vi "Get Semaphore.vi"(4 "error in":errorcluster, 7 "VISA In":refnum<visa-resource-name>) -> (0 "error out":errorcluster, 2 "semaphore out":T1, 3 "VISA Out":refnum<visa-resource-name>)   [LabVIEW 2020]
doc: "Developed by Kevin Thompson\nkevin@thompsonengineering.net\n\nCopyright 2018-2020\nThompson Engineering, LLC"
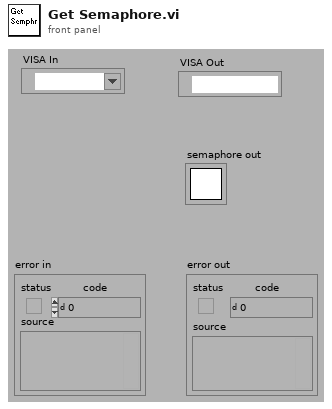
[diagram p1: front panel]
types:
  T1 = typedef "Semaphore RefNum" = refnum<k1>
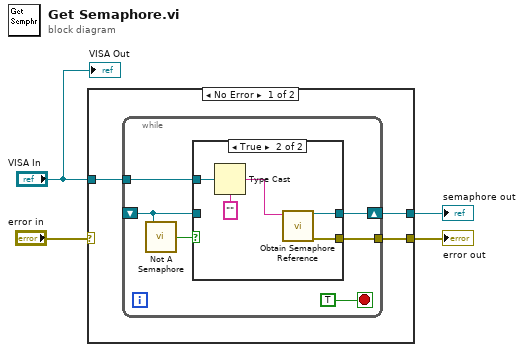
[diagram p0: block diagram]
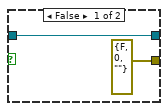
[diagram p2: hidden frame]
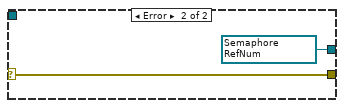
[diagram p3: hidden frame]
diagram:
  n1 = case shown="No Error" "error in" {
    selector: "error in" -> [_ w22]
    tunnel: "VISA In" -> [w7 _]
    tunnel: [w6 w21] -> w2
    tunnel: [w5 w22] -> w3
    frame No Error {
      n2 = while {
        shift-right: [w11] -> w6
        shift-left: _ -> [w12]
        tunnel: w7 -> [w10]
        tunnel: [w8] -> w5
        stop <- TRUE stop-if-true
        n3 = call <vilib>:"Not A Semaphore.vi"("semaphore"=w12) -> ("not a semaphore"=w13:bool)
        n4 = case shown="True" w13 {
          tunnel: w12 -> [w15 _]
          tunnel: [w15 w20] -> w11
          tunnel: w10 -> [_ w19]
          tunnel: [errorcluster {"status"=FALSE, "code"=0, "source"=""} ("error out") w16] -> w8
          frame False {
          }
          frame True {
            n5 = Type Cast(type="", x=w19) -> (*(type *) &x=w17:string)
            n6 = call <vilib>:"Obtain Semaphore Reference.vi"("name (unnamed)"=w17) -> ("error out"=w16:errorcluster, "semaphore"=w20:T1)  [unwired: 4 in, 1 out]
          }
        }
      }
    }
    frame Error {
      w21 = T1 refnum items=["semaphore"] ("semaphore")
    }
  }
  "error out" <- w3
  "semaphore out" <- w2
  "VISA Out" <- "VISA In"
